vi "Generate Random GBs.vi"() -> ()   [LabVIEW 2010]
uses:
  <vilib>/Utility/file.llb/Write To Spreadsheet File (string).vi
panel:
  in  "How many to make?":i32=10000
  out "GBs to make":T1(array[cluster])
  in  "Path":path
  in  "Reduce to Repeating":T2={"Slab X"=4.6, "Slab Y"=4.0, "Tolerance (A)"=0.5, "Presorted?"=FALSE}
  out "Current Index":i32
  in  "Relaxation Type":string(combo)="conp opti"
  out "# of Reduced":i32
  in  "Grain Growth and Geometry":T3={"Grain 1 Length (prop)"=1.0, "Grain 2 Length (prop)"=1.0, "Max Grain Height (A)"=80.0, "Max Grain Width (A)"=80.0, "Grain 1 Start"=-0.001, "Overlap Region (A)"=0.001}
  out "Numeric":i32
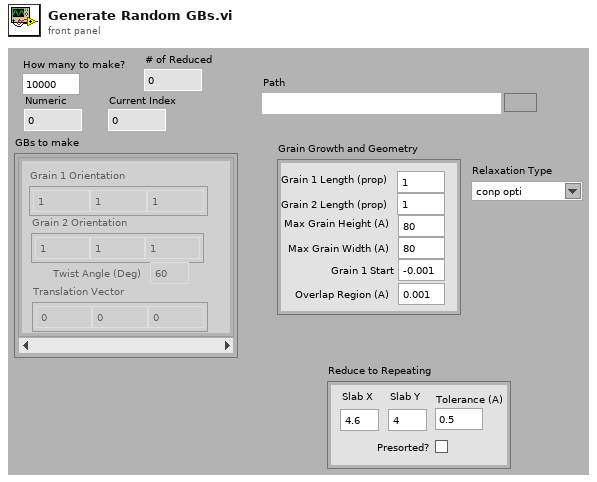
[diagram p1: front panel]
types:
  T1 = cluster{"Grain 1 Orientation":dbl[], "Grain 2 Orientation":dbl[], "Twist Angle (Deg)":dbl, "Translation Vector":dbl[]}[]
  T2 = cluster{"Slab X":dbl, "Slab Y":dbl, "Tolerance (A)":dbl, "Presorted?":bool}
  T3 = cluster{"Grain 1 Length (prop)":dbl, "Grain 2 Length (prop)":dbl, "Max Grain Height (A)":dbl, "Max Grain Width (A)":dbl, "Grain 1 Start":dbl, "Overlap Region (A)":dbl}
  T4 = cluster{"Grain 1 Orientation":dbl[], "Grain 2 Orientation":dbl[], "Twist Angle (Deg)":dbl, "Grain 2 Orientation 2":dbl[]}
  T5 = cluster{"Grain 1 Orientation":dbl[], "Grain 2 Orientation":dbl[], "Twist Angle (Deg)":dbl, "Grain 2 Orientation 2":dbl[]}[]
  T6 = cluster{"Structure Name":string, "Lattice vector a":dbl[], "Lattice vector b":dbl[], "Lattice vector c":dbl[], "Atoms Array":cluster{"Atom Name":string, "Positions (Direct)":dbl[][], "Positions (Cartesian)":dbl[][]}[], "# of atoms":i32}
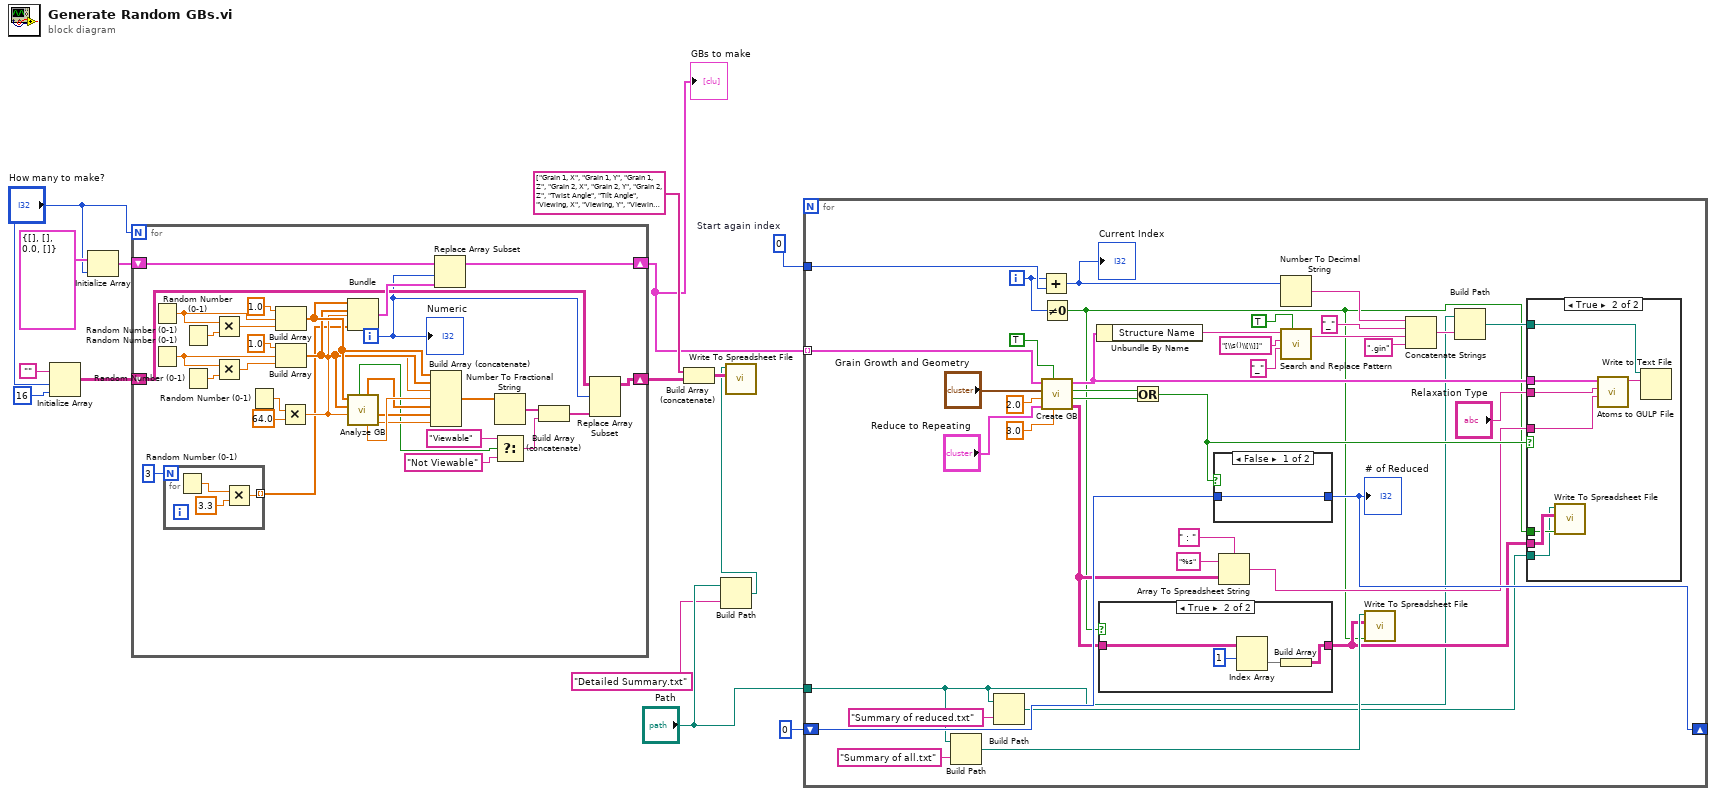
[diagram p0: block diagram]
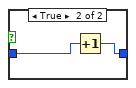
[diagram p4: hidden frame]
diagram:
  w5 = 0  # Start again index
  n1 = Initialize Array("", "How many to make?", 16 ("dimension size")) -> (w10:string[][])
  n2 = Initialize Array(T4 {"Grain 1 Orientation"=[], "Grain 2 Orientation"=[], "Twist Angle (Deg)"=0.0, "Grain 2 Orientation 2"=[]} ("Grain Boundary Definition"), "How many to make?") -> (w14:T5)
  n3 = for {
    N: "How many to make?" -> [_]
    shift-right: [w35] -> w4
    shift-left: w14 -> [w37]
    shift-right: [w29] -> w7
    shift-left: w10 -> [w31]
    i -> [w30]
    n4 = Random Number (0-1)() -> (number: 0 to 1=w46:dbl)
    n5 = Random Number (0-1)() -> (number: 0 to 1=w42:dbl)
    n6 = for {
      N: 3 -> [_]
      tunnel: [w48] -> w17 mode=indexing
      n7 = Random Number (0-1)() -> (number: 0 to 1=w50:dbl)
      n8 = Multiply(x=w50, y=3.3) -> (x*y=w48:dbl)
    }
    n9 = Random Number (0-1)() -> (number: 0 to 1=w47:dbl)
    n10 = Random Number (0-1)() -> (number: 0 to 1=w41:dbl)
    n11 = Multiply(x=w46, y=w47) -> (x*y=w45:dbl)
    n12 = Multiply(x=w42, y=w41) -> (x*y=w40:dbl)
    n13 = Random Number (0-1)() -> (number: 0 to 1=w39:dbl)
    n14 = Build Array(1.0 ("element"), w46, w45) -> (w27:dbl[])
    n15 = Build Array(1.0 ("element"), w42, w40) -> (w26:dbl[])
    n16 = Multiply(x=w39, y=64.0) -> (x*y=w25:dbl)
    n17 = Bundle(w27, w26, w25, w17) -> (w36:cluster{dbl[], dbl[], dbl, dbl[]})  [unwired: 1 in]
    n18 = call "Analyze GB.vi"("Twist Angle (Deg)"=w25, "Grain 2 Orientation"=w26, "Grain 1 Orientation"=w27) -> ("Misorientation Angle"=w32:dbl, "Misorientation Axis, o"=w33:dbl[], "Tilt Angle (Deg)"=w34:dbl, "Suggested Viewing Angle"=w24:dbl[], "Viewable?"=w23:bool)  [unwired: 1 in, 3 out]
    n19 = Build Array (concatenate)(w27, w26, w25, w34, w24, w33, w32) -> (w28:dbl[])
    n20 = Replace Array Subset(array=w37, new element=w36, index=w30) -> (w35:T5)
    n21 = Number To Fractional String(number=w28) -> (F-format string=w21:string[])  [unwired: 3 in]
    n22 = Select(t="Viewable", s=w23, f="Not Viewable") -> (s? t:f=w20:string)
    n23 = Build Array (concatenate)(w21, w20) -> (w19:string[])
    n24 = Replace Array Subset(array=w31, new element=w19, index (row)=w30) -> (w29:string[][])  [unwired: 1 in]
    "Numeric" <- w30
  }
  "GBs to make" <- w4
  n25 = Build Array (concatenate)(string[] ["Grain 1, X", "Grain 1, Y", "Grain 1, Z", "Grain 2, X", "Grain 2, Y", "Grain 2, Z", "Twist Angle", "Tilt Angle", "Viewing, X", "Viewing, Y", "Viewing, Z", "Mis, X", "Mis, Y", "Mis, Z", "Mis Angle", "Viewable"] ("Data 2"), w7) -> (w9:string[][])
  n26 = Build Path(base path="Path", name or relative path="Detailed Summary.txt") -> (appended path=w1:path)
  n27 = call-poly <vilib>:"Write To Spreadsheet File.vi"("2D data"=w9, "file path (dialog if empty)"=w1) -> ()  [unwired: 6 in, 1 out]
  n28 = for {
    tunnel: "Path" -> [w54]
    shift-right: [w70] -> _
    shift-left: 0 -> [w71]
    tunnel: w4 -> [w67] mode=indexing
    tunnel: w5 -> [w66]
    i -> [w59]
    n29 = Build Path(base path=w54, name or relative path="Summary of all.txt") -> (appended path=w58:path)
    n30 = Build Path(base path=w54, name or relative path="Summary of reduced.txt") -> (appended path=w52:path)
    n31 = Add(x=w59, y=w66) -> (x+y=w65:i32)
    "Current Index" <- w65
    n32 = Not Equal To 0?(x=w59) -> (x != 0?=w55:bool)
    n33 = call "Create GB.vi"("Edge Duplication Range"=3.0, "Skip cleanup if no subset"=TRUE ("Skip crop if no subset"), "Reduce to Repeating"="Reduce to Repeating", "Min Seperation Distance (A)"=2.0, "Grain Growth and Geometry"="Grain Growth and Geometry", "Grain Boundary Definition"=w67) -> ("GB Data"=w57:string[][], "Reduced Orthorhombic?"=w72:bool, "Reduced Rhombahedral?"=w73:bool, "Grain Boundary"=w87:T6)  [unwired: 1 in, 1 out]
    n34 = Unbundle By Name(w87) -> ("Structure Name"=w76:string)
    n35 = case shown="True" w55 {
      tunnel: [w88 w89] -> w56
      tunnel: w57 -> [w88 w92]
      frame False {
      }
      frame True {
        n36 = Index Array(array=w92, index (row)=1) -> (element=w90:string[])  [unwired: 1 in]
        n37 = Build Array(w90) -> (w89:string[][])
      }
    }
    n38 = Or(x=w73, y=w72) -> (x .or. y?=w69:bool)
    n39 = case shown="False" w69 {
      tunnel: w71 -> [w101 w103]
      tunnel: [w101 w102] -> w70
      frame False {
      }
      frame True {
        n40 = Increment(x=w103) -> (x+1=w102:i32)
      }
    }
    "# of Reduced" <- w70
    n41 = Array To Spreadsheet String(delimiter (Tab)=" : ", array=w57, 3:"%s" ("format string")) -> (spreadsheet string=w61:string)
    n42 = Number To Decimal String(number=w65) -> (decimal integer string=w86:string)  [unwired: 1 in]
    n43 = call <vilib>:"Search and Replace Pattern.vi"("string"=w76, "regular expression (\"\")"="[\\s()\\[\\]]" ("regular expression (\"\")"), "replace string (\"\")"="_" ("replace string (\"\")"), "replace all? (F)"=TRUE) -> ("result string"=w75:string)  [unwired: 1 in, 1 out]
    n44 = call-poly <vilib>:"Write To Spreadsheet File.vi"("append to file? (new file:F)"=w55, "2D data"=w56, "file path (dialog if empty)"=w58) -> ()  [unwired: 5 in, 1 out]
    n45 = Concatenate Strings(w86, "_" ("string"), w75, ".gin" ("string")) -> (w85:string)
    n46 = Build Path(base path=w54, name or relative path=w85) -> (appended path=w84:path)
    n47 = case shown="True" w69 {
      tunnel: w87 -> [_ w100]
      tunnel: w84 -> [_ w99]
      tunnel: "Relaxation Type" -> [_ w98]
      tunnel: w61 -> [_ w96]
      tunnel: w56 -> [_ w95]
      tunnel: w55 -> [_ w94]
      tunnel: w52 -> [_ w93]
      frame False {
      }
      frame True {
        n48 = call-poly <vilib>:"Write To Spreadsheet File.vi"("append to file? (new file:F)"=w94, "2D data"=w95, "file path (dialog if empty)"=w93) -> ()  [unwired: 5 in, 1 out]
        n49 = call "Atoms to GULP File.vi"("Title and Comments"=w96, "Relaxation Type"=w98, "Structure"=w100) -> ("GULP File"=w97:string)  [unwired: 8 in]
        n50 = Write to Text File(file (use dialog)=w99, text=w97) -> ()  [unwired: 2 in, 3 out]
      }
    }
  }
